vi "HexStringToSample.vi"(11 "StringIn":string) -> (0 "ErrorOut":errorcluster, 2 "StringOut":string, 3 "Sample":T1)   [LabVIEW 2016]
doc: "Convert string to measurement data."
uses:
  FallSensor/Sample.ctl
  FallSensor/Reading.ctl
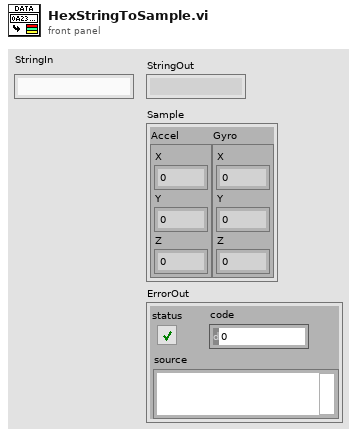
[diagram p1: front panel]
types:
  T1 = typedef "Sample.ctl" = cluster{"Accel":T2, "Gyro":T2}
  T2 = typedef "Reading.ctl" = cluster{"X":dbl, "Y":dbl, "Z":dbl}
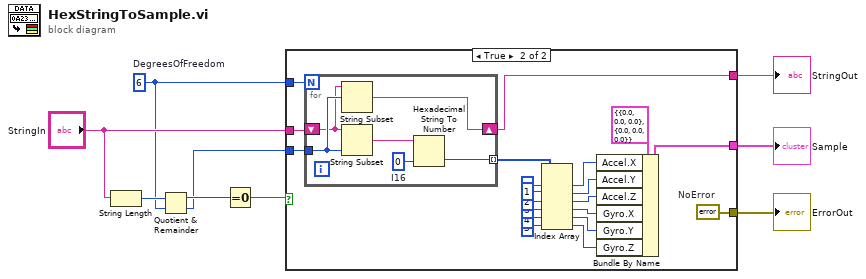
[diagram p0: block diagram]
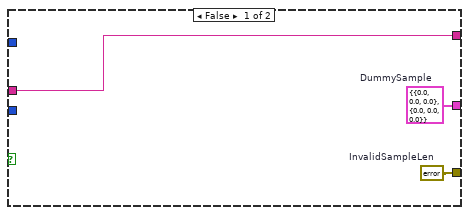
[diagram p2: hidden frame]
diagram:
  w3 = 6  # DegreesOfFreedom
  n1 = String Length(string="StringIn") -> (length=w9:i32)
  n2 = Quotient & Remainder(x=w9, y=w3) -> (x-y*floor(x/y)=w8:i32, floor(x/y)=w4:i32)
  n3 = Equal To 0?(x=w8) -> (x = 0?=w7:bool)
  n4 = case shown="True" w7 {
    tunnel: [w12 w32] -> w6
    tunnel: "StringIn" -> [w10 w30]
    tunnel: w4 -> [_ w29]
    tunnel: w3 -> [_ w31]
    tunnel: [w11 w14] -> w1
    tunnel: [w10 w15] -> w2
    frame False {
      w11 = T1 {"Accel"={"X"=0.0, "Y"=0.0, "Z"=0.0}, "Gyro"={"X"=0.0, "Y"=0.0, "Z"=0.0}}  # DummySample
      w12 = errorcluster {"status"=TRUE, "code"=4, "source"="Invalid sample length"}  # InvalidSampleLen
    }
    frame True {
      w32 = errorcluster {"status"=FALSE, "code"=0, "source"=""}  # NoError
      n5 = for {
        N: w31 -> [_]
        shift-right: [w37] -> w15
        shift-left: w30 -> [w35]
        tunnel: w29 -> [w36]
        tunnel: [w33] -> w28 mode=indexing
        w34 = i16 0  # I16
        n6 = String Subset(string=w35, offset (0)=w36) -> (substring=w37:string)  [unwired: 1 in]
        n7 = String Subset(string=w35, length (rest)=w36) -> (substring=w38:string)  [unwired: 1 in]
        n8 = Hexadecimal String To Number(string=w38, default (0uL)=w34) -> (number=w33:i16)  [unwired: 1 in, 1 out]
      }
      n9 = Index Array(array=w28, index #1=0 ("index"), index #2=1 ("index"), index #3=2 ("index"), index #4=3 ("index"), index #5=4 ("index"), index #6=5 ("index")) -> (element #1=w21:i16, element #2=w20:i16, element #3=w19:i16, element #4=w18:i16, element #5=w17:i16, element #6=w16:i16)
      n10 = Bundle By Name(cluster=T1 {"Accel"={"X"=0.0, "Y"=0.0, "Z"=0.0}, "Gyro"={"X"=0.0, "Y"=0.0, "Z"=0.0}} ("Sample"), "Accel.X"=w21, "Accel.Y"=w20, "Accel.Z"=w19, "Gyro.X"=w18, "Gyro.Y"=w17, "Gyro.Z"=w16) -> (w14:T1)
    }
  }
  "ErrorOut" <- w6
  "StringOut" <- w2
  "Sample" <- w1
